vi "Get_picture_size_test.vi"() -> ()   [LabVIEW 2020]
uses:
  <vilib>/Utility/miscctls.llb/LVBoundsTypeDef.ctl
panel:
  out "error out":errorcluster
  in  "error in (no error)":errorcluster
  out "Draw Area Size":T1
  in  "Path":path
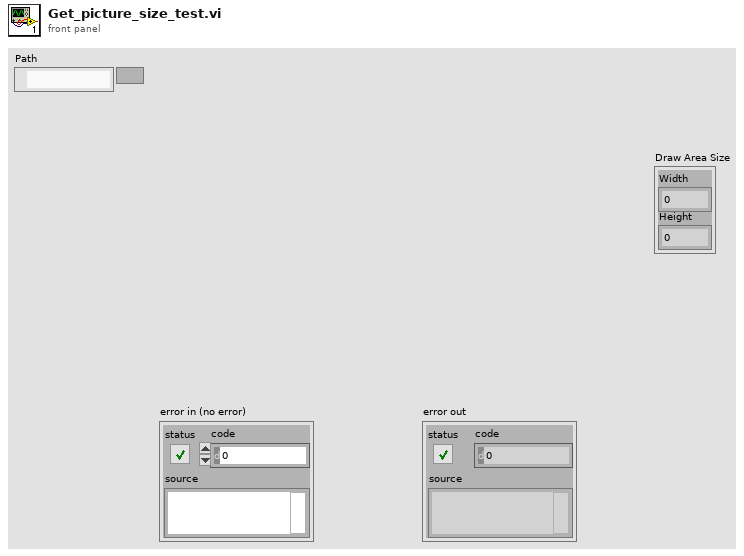
[diagram p1: front panel]
types:
  T1 = typedef "LVBoundsTypeDef.ctl" = cluster{"Width":u32, "Height":u32}
  T2 = typedef "imagedata.ctl" = cluster{"image type":i32, "image depth":i32, "image":u8[], "mask":u8[], "colors":u32[], "Rectangle":cluster{"left":i16, "top":i16, "right":i16, "bottom":i16}}
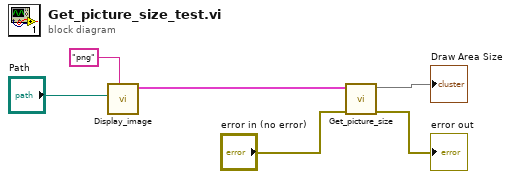
[diagram p0: block diagram]
diagram:
  n1 = call "Display_image.vi"("lowercase file extension"="png", "path file"="Path") -> ("image data"=w4:T2)  [unwired: 7 in, 2 out]
  n2 = call "Get_picture_size.vi"("error in (no error)"="error in (no error)", 11:w4) -> ("error out"=→"error out":errorcluster, 3:→"Draw Area Size")  [unwired: 7 in, 1 out]
